vi "Timescale_Factor.vi"(0 "Integration threshold (0...1)_":dbl=0.1, 1 "Timescale scaling factor_":dbl=1.12) -> (2 "Integration threshold (0...1)":dbl, 3 "Timescale scaling factor":dbl=1.0, 4 "Multiplyer of Timescale to get Independant samples":dbl=2.0)   [LabVIEW 2016]
panel:
  # "This is the fraction of the correlation peak value at which to cut-off the integration of the correlation function"
  # "Set values as default to make permanent changes"
  # "This if the factor to multiply the integral time scale by to correct for a non-zero integration cut-off"
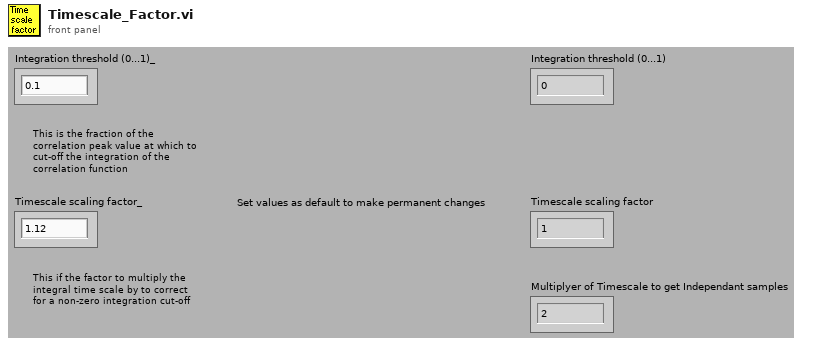
[diagram p1: front panel]
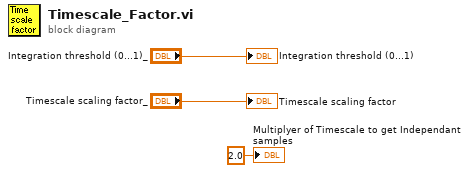
[diagram p0: block diagram]
diagram:
  "Integration threshold (0...1)" <- "Integration threshold (0...1)_"
  "Timescale scaling factor" <- "Timescale scaling factor_"
  "Multiplyer of Timescale to get Independant samples" <- 2.0 ("Multiplyer of Timescale to get Independant samples")
